vi "Define_Point_Category_for_Status_Matrix-1.vi"(0 "[IN] Summarized\npoint status":i16) -> (1 "[OUT] Point isn't \nlabeled with \"10\"":bool, 2 "[OUT] Category of point":u8, 3 "[OUT] Point isn't \nlabeled with \"100\"":bool)   [LabVIEW 2013]
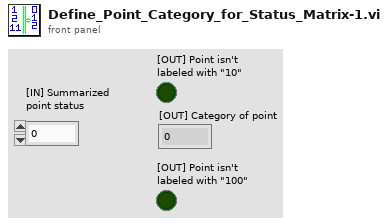
[diagram p1: front panel]
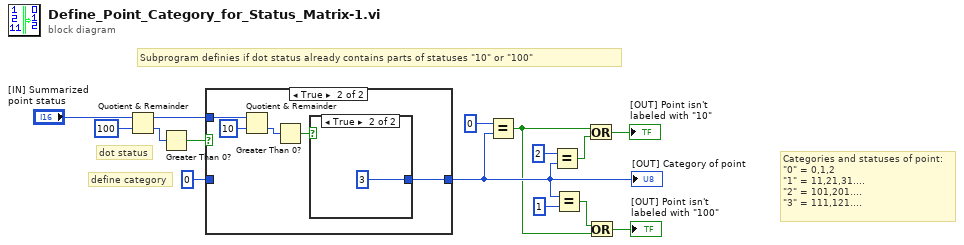
[diagram p0: block diagram]
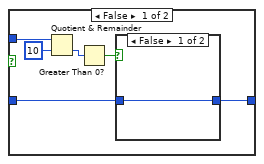
[diagram p2: hidden frame]
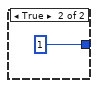
[diagram p3: hidden frame]
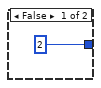
[diagram p4: hidden frame]
diagram:
  # "define category"
  # "Subprogram definies if dot status already contains parts of statuses \"10\" or \"100\""
  # "Categories and statuses of point:\n\"0\" = 0,1,2\n\"1\" = 11,21,31....\n\"2\" = 101,201....\n\"3\" = 111,121...."
  # "dot status"
  n1 = Quotient & Remainder(x="[IN] Summarized\npoint status", y=i16 100) -> (x-y*floor(x/y)=w15:i16, floor(x/y)=w12:i16)
  n2 = Greater Than 0?(x=w12) -> (x > 0?=w13:bool)
  n3 = case shown="True" w13 {
    tunnel: u8 0 -> [w17 _]
    tunnel: w15 -> [w19 w28]
    tunnel: [w16 w24] -> w4
    frame False {
      n4 = Quotient & Remainder(x=w19, y=i16 10) -> (floor(x/y)=w20:i16)  [unwired: 1 out]
      n5 = Greater Than 0?(x=w20) -> (x > 0?=w18:bool)
      n6 = case shown="False" w18 {
        tunnel: w17 -> [w22 _]
        tunnel: [w22 u8 1] -> w16
        frame False {
        }
        frame True {
        }
      }
    }
    frame True {
      n7 = Quotient & Remainder(x=w28, y=i16 10) -> (floor(x/y)=w26:i16)  [unwired: 1 out]
      n8 = Greater Than 0?(x=w26) -> (x > 0?=w25:bool)
      n9 = case shown="True" w25 {
        tunnel: [u8 2 u8 3] -> w24
        frame False {
        }
        frame True {
        }
      }
    }
  }
  "[OUT] Category of point" <- w4
  n10 = Equal?(x=u8 0, y=w4) -> (x = y?=w2:bool)
  n11 = Equal?(x=u8 2, y=w4) -> (x = y?=w8:bool)
  n12 = Equal?(x=w4, y=u8 1 ("x")) -> (x = y?=w3:bool)
  n13 = Or(x=w2, y=w8) -> (x .or. y?=→"[OUT] Point isn't \nlabeled with \"10\"":bool)
  n14 = Or(x=w3, y=w2) -> (x .or. y?=→"[OUT] Point isn't \nlabeled with \"100\"":bool)
